vi "Close Instrument.vi"(8 "error in (no error)":errorcluster, 11 "Simulated Sig Gen.lvclass in":refnum<class "Simulated Sig Gen.lvclass">) -> (0 "error out":errorcluster, 3 "Simulated Sig Gen.lvclass out":refnum<class "Simulated Sig Gen.lvclass">)   [LabVIEW 2010, in "Simulated Sig Gen.lvclass"]
uses:
  Simulated Sig Gen.lvclass
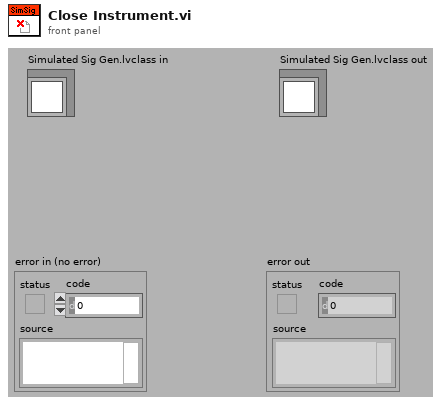
[diagram p1: front panel]
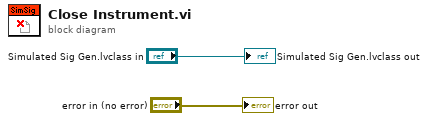
[diagram p0: block diagram]
diagram:
  "error out" <- "error in (no error)"
  "Simulated Sig Gen.lvclass out" <- "Simulated Sig Gen.lvclass in"
